vi "Gmsg_RR_Pinger.vi"() -> ()   [LabVIEW 2013]
uses:
  Actor/src/Client/FTW-Client.lvclass
  <vilib>/ptbypt/NI_PtbyPt.lvlib
panel:
  out "Average Roundtrip Time":dbl format="%.6fsec"
  out "Roundtrip Time Chart":cluster{"Roundtrip Time":dbl, "mean":dbl}(graph)
  in  "Ping Rate":i32=500
  out "Roundtrip Time":dbl format="%.6fsec"
  in  "Connection":string(combo)="lvq://someLVQconnection"
  out "Connected":bool
  in  "Ask Timeout":i32=1000
  out "Response Body":string
  in  "Message Size":i32=1
  out "Response Header":string
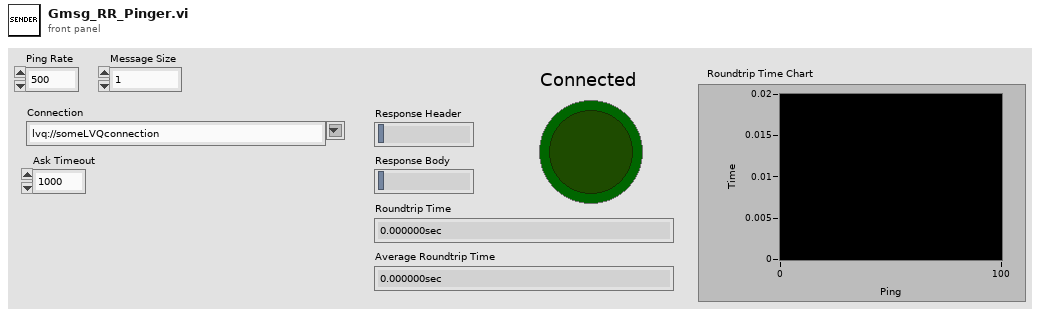
[diagram p1: front panel]
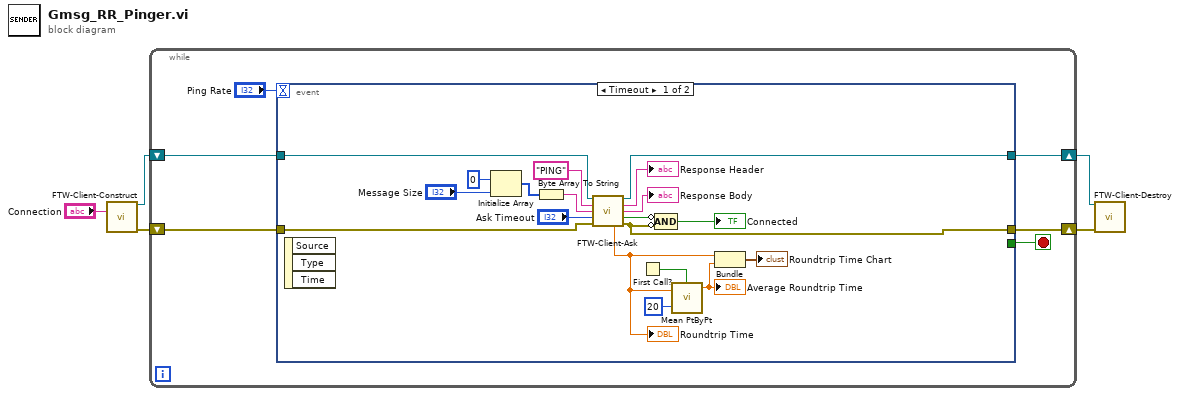
[diagram p0: block diagram]
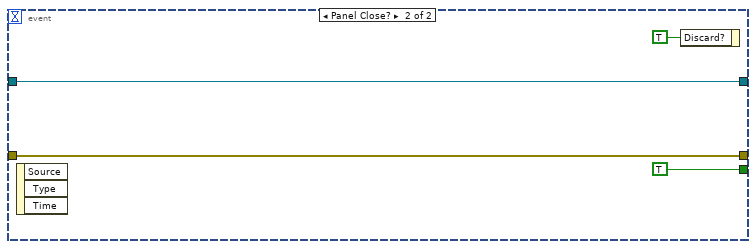
[diagram p2: hidden frame]
diagram:
  n1 = call "FTW-Client-Construct.vi"("Server Address"="Connection") -> ("FTW-Client Out"=w4:refnum<class "FTW-Client.lvclass">, "error out"=w3:errorcluster)  [unwired: 13 in]
  n2 = while {
    shift-right: [w8] -> w1
    shift-left: w4 -> [w9]
    shift-right: [w6] -> w2
    shift-left: w3 -> [w7]
    stop <- w11 stop-if-true
    n3 = event shown="[0] Timeout" {
      selector: _ -> [_ _]
      dyn-events: _ -> [_ _]
      timeout: "Ping Rate" -> [_ _]
      tunnel: [_ TRUE ("Discard?")] -> w11
      tunnel: w9 -> [w30 w32]
      tunnel: [w29 w32] -> w8
      tunnel: w7 -> [w28 w31]
      tunnel: [w19 w31] -> w6
      event Timeout {
        n4 = event-data() -> ()  [unwired: 1 in, 3 out]
        n5 = Initialize Array(u8 0, "Message Size") -> (w24:u8[])
        n6 = Byte Array To String(unsigned byte array=w24) -> (string=w21:string)
        n7 = call "FTW-Client-Ask.vi"("FTW-Client In"=w30, "Header"="PING", "Body"=w21, "Timeout"="Ask Timeout", "error in"=w28) -> ("FTW-Client Out"=w29:refnum<class "FTW-Client.lvclass">, "Response Header"=→"Response Header":string, "Response Body"=→"Response Body":string, "Timed out?"=w18:bool, "Roundtrip Time"=w15:dbl, "error out"=w19:errorcluster)  [unwired: 5 in]
        "Roundtrip Time" <- w15
        n8 = First Call?() -> (First Call?: T/F=w16:bool)
        n9 = Compound Arithmetic op=AND(invert w18, invert w19) -> (→"Connected":bool)
        n10 = call <vilib>:"Mean PtByPt.vi"("x"=w15, "sample length"=20, "initialize"=w16) -> ("mean"=w13:dbl)  [unwired: 1 in, 1 out]
        "Average Roundtrip Time" <- w13
        n11 = Bundle("Roundtrip Time"=w15, "mean"=w13) -> (→"Roundtrip Time Chart":cluster{"Roundtrip Time":dbl, "mean":dbl})  [unwired: 1 in]
      }
      event Panel Close? {
        n12 = event-data() -> ()  [unwired: 1 in, 3 out]
        n13 = event-data("Discard?"=TRUE) -> ()  [unwired: 1 in, 1 out]
      }
    }
  }
  n14 = call "FTW-Client-Destroy.vi"("FTW-Client In"=w1, "error in"=w2) -> ()  [unwired: 13 in, 1 out]
